vi "dfd_CIC_Decimator.vi"(10 "input valid":bool=TRUE, 11 "input data":bool[](array[boolean])) -> (0 "ready for input":bool, 2 "output valid":bool, 3 "output data":bool[](array[boolean]))   [LabVIEW 2017]
uses:
  <vilib>/rvi/FXPMathLib/basic elements/FxpDiscreteDelay/XNode/nifxpmath_DiscreteDelay.xnode
  <vilib>/rvi/FXPMathLib/basic elements/FxpAddSub/XNode/nifxpmath_AddSub.xnode
  <vilib>/rvi/FXPMathLib/sim/FxpSim.dll
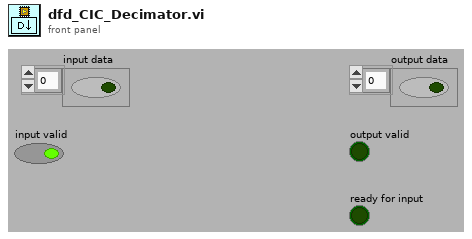
[diagram p1: front panel]
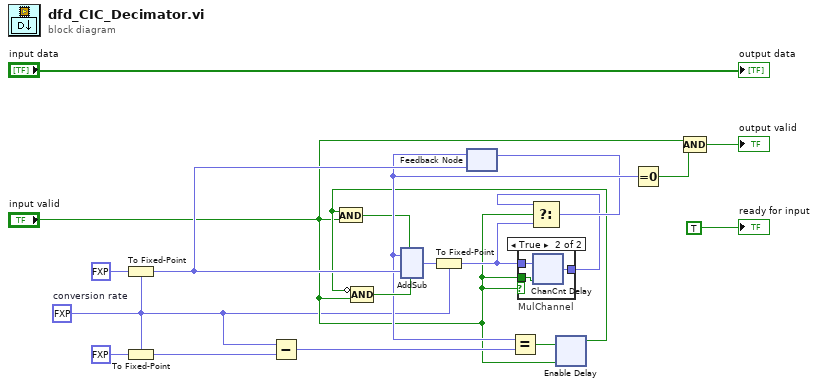
[diagram p0: block diagram]
diagram:
  w1 = fxp<+,2,2> 3.0  # conversion rate
  n1 = To Fixed-Point(fixed-point type=w1, number=fxp<+,2,2> 0.0 ("fixed-point")) -> (fixed-point=w20:fxp<+,2,2>)
  n2 = To Fixed-Point(fixed-point type=w1, number=fxp<+,2,2> 2.0 ("fixed-point")) -> (fixed-point=w19:fxp<+,2,2>)
  n3 = Subtract(x=w1, y=w19) -> (x-y=w18:fxp<+/-,3,3>)
  n4 = feedback #1(w20) -> (w16:fxp<+,2,2>)
  n5 = Equal?(x=w16, y=w18) -> (x = y?=w9:bool)
  n6 = xnode "Enable Delay"("D"=w9, "enable"="input valid") -> ("Q"=w8:bool)
  n7 = And(x=w8, y="input valid") -> (x .and. y?=w12:bool)
  n8 = Compound Arithmetic op=AND(invert w8, "input valid") -> (w17:bool)
  n9 = xnode ("AddSub")("x"=w16, "y"=w20, "carry-in"=w17, "use zero instead of x"=w12) -> ("s"=w11:fxp<+,2,2>)  [unwired: 1 out]
  n10 = To Fixed-Point(fixed-point type=w1, number=w11) -> (fixed-point=w10:fxp<+,2,2>)
  n11 = case "MulChannel" shown="True" "input valid" {
    tunnel: [w21 w24] -> w13
    tunnel: w10 -> [w21 w23]
    tunnel: "input valid" -> [_ w22]
    frame False {
    }
    frame True {
      n12 = xnode ("ChanCnt Delay")("D"=w23, "enable"=w22) -> ("Q"=w24:fxp<+,2,2>)
    }
  }
  n13 = Select(t=w13, s="input valid", f=w10) -> (s? t:f=w14:fxp<+,2,2>)
  n14 = feedback-in #1(w14) -> ()
  n15 = Equal To 0?(x=w16) -> (x = 0?=w15:bool)
  n16 = Compound Arithmetic op=AND("input valid", w15) -> (→"output valid":bool)
  "ready for input" <- TRUE
  "output data" <- "input data"
